vi "Read Packet Type.vi"(8 "error in (no error)":errorcluster, 11 "JSONPayload in":refnum<class "JSONPayload.lvclass">) -> (0 "error out":errorcluster, 2 "Packet Type":string, 3 "JSONPayload out":refnum<class "JSONPayload.lvclass">)   [LabVIEW 2019, in "JSONPayload.lvclass"]
uses:
  JSONPayload.lvclass
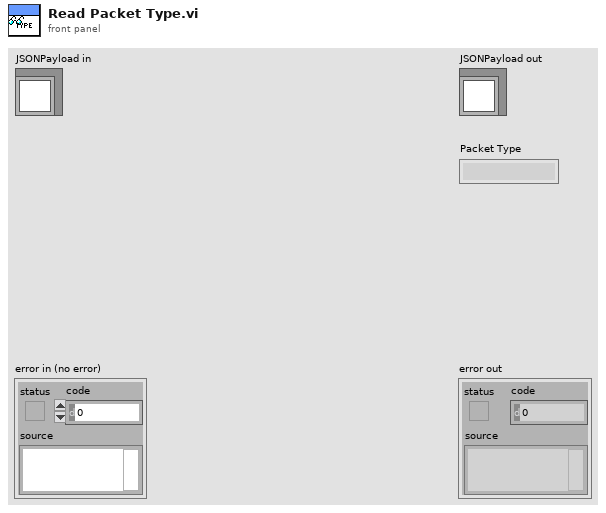
[diagram p1: front panel]
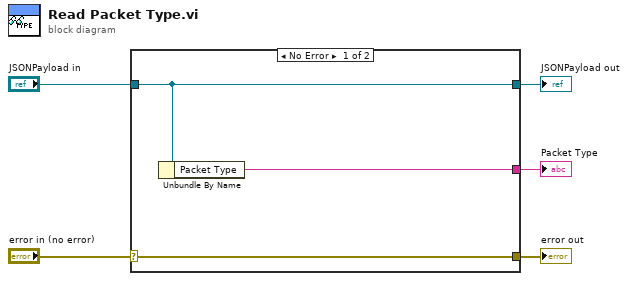
[diagram p0: block diagram]
diagram:
  n1 = case shown="No Error" "error in (no error)" {
    selector: "error in (no error)" -> [w8 w9]
    tunnel: [w8 w9] -> w4
    tunnel: [w7 w10] -> w2
    tunnel: "JSONPayload in" -> [w7 w10]
    tunnel: [w6 _] -> w1
    frame No Error {
      n2 = Unbundle By Name(w7) -> ("Packet Type"=w6:string)
    }
    frame Error {
    }
  }
  "error out" <- w4
  "JSONPayload out" <- w2
  "Packet Type" <- w1
